vi "Goto Point.vi"(0 "Target X (Relative)":dbl=200.0, 1 "Target Y (Relative)":dbl, 2 "Bot Angle":dbl=6.265957027809849, 3 "dt":dbl=0.03, 5 "Stop motors":bool, 6 "Speed":T1={"\nMoving speed"=1.0296610169491527, "Turning speed limit"=1.0169491525423728} {"Turning speed limit" scale=0.0..4.5; "Moving speed" scale=0.0..1.0}) -> ()   [LabVIEW 2017]
uses:
  <vilib>/addons/control/pid/pid.llb/PID (DBL).vi
  Globals/Motor Speed Multiplier.vi
  <vilib>/addons/control/pid/NI_PID_pid.lvlib
panel:
  in  "Turning PID":cluster{"P":dbl, "I":dbl, "D":dbl}={"P"=-0.4, "I"=0.0, "D"=0.003}
  in  "threshold angle":dbl=0.3
  out "Right motor speed":dbl=0.013786667806161291
  out "Left motor speed":dbl=-0.013786667806161291
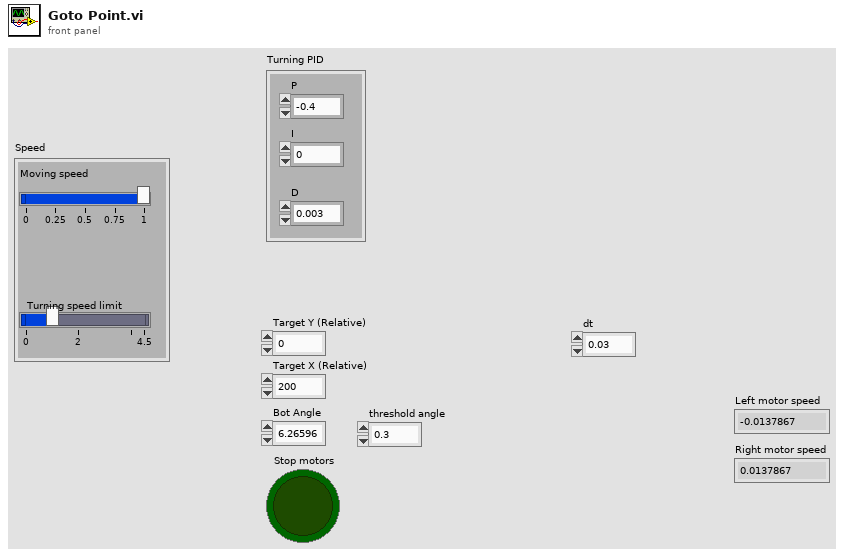
[diagram p1: front panel]
types:
  T1 = cluster{"\nMoving speed":dbl, "Turning speed limit":dbl}
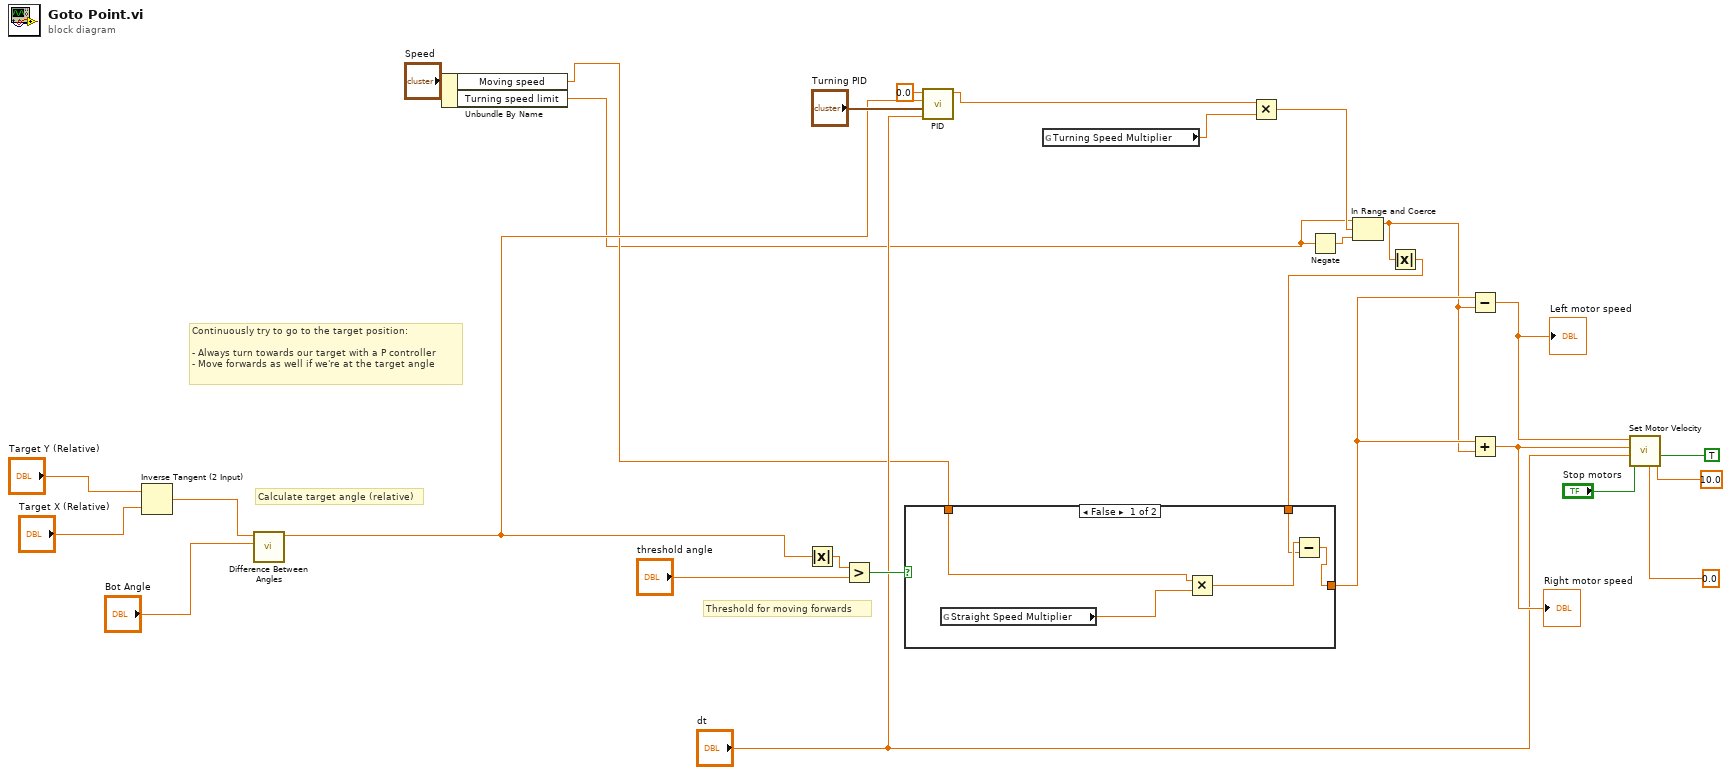
[diagram p0: block diagram]
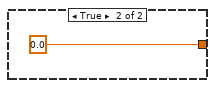
[diagram p2: hidden frame]
diagram:
  # "Threshold for moving forwards"
  # "Calculate target angle (relative)"
  # "Continuously try to go to the target position:\n\n- Always turn towards our target with a P controller\n- Move forwards as well if we're at the target angle"
  n1 = Inverse Tangent (2 Input)(1:"Target X (Relative)", 2:"Target Y (Relative)") -> (0:w26:dbl)
  n2 = call "Difference Between Angles.vi"("Angle 2"="Bot Angle", "Angle 1"=w26) -> ("Difference"=w7:dbl)  [unwired: 9 in]
  n3 = Unbundle By Name("Speed") -> ("Moving speed"=w4:dbl, "Turning speed limit"=w3:dbl)
  n4 = Absolute Value(x=w7) -> (abs(x)=w19:dbl)
  n5 = Greater?(x=w19, y="threshold angle") -> (0:w15:bool)
  n6 = call-poly <vilib>:"PID.vi"("dt (s)"="dt", "PID gains"="Turning PID", "process variable"=w7, "setpoint"=0.0) -> ("output"=w2:dbl)  [unwired: 6 in, 1 out]
  n7 = global read "Motor Speed Multiplier.vi" "Turning Speed Multiplier"() -> (w1:dbl)
  n8 = Multiply(x=w2, y=w1) -> (x*y=w13:dbl)
  n9 = Negate(x=w3) -> (-x=w12:dbl)
  n10 = In Range and Coerce(upper limit=w3, x=w13, lower limit=w12) -> (coerced(x)=w11:dbl)  [unwired: 1 out]
  n11 = Absolute Value(x=w11) -> (abs(x)=w10:dbl)
  n12 = case shown="False" w15 {
    tunnel: [w29 0.0] -> w16
    tunnel: w10 -> [w30 _]
    tunnel: w4 -> [w28 _]
    frame False {
      n13 = global read "Motor Speed Multiplier.vi" "Straight Speed Multiplier"() -> (w32:dbl)
      n14 = Multiply(x=w28, y=w32) -> (x*y=w31:dbl)
      n15 = Subtract(x=w31, y=w30) -> (x-y=w29:dbl)
    }
    frame True {
    }
  }
  n16 = Subtract(x=w16, y=w11) -> (x-y=w17:dbl)
  "Left motor speed" <- w17
  n17 = Add(x=w16, y=w11) -> (x+y=w18:dbl)
  "Right motor speed" <- w18
  n18 = call "Set Motor Velocity.vi"("Acceleration ramp constant"=10.0, "Accelerate?"=TRUE, "Back motor speed rev/s"=0.0 ("result"), "Disable motors"="Stop motors", "dt"="dt", "Right motor speed rev/s"=w18, "Left motor speed rev/s"=w17) -> ()  [unwired: 5 in]
